vi "Main Engine.vi"(8 "error in":errorcluster) -> (0 "error out":errorcluster)   [LabVIEW 2021]
doc: "This VI will launch all engines handle and close all references.\n\n\n\nAll Rights Reserved © 2023 SyncSols"
uses:
  Controls/Main Engine State Machine Data Cluster.ctl
  Controls/Main Engine Hardware Info Data Cluster.ctl
  Controls/Main Engine DAQ Device Info.ctl
  Controls/Main Engine Serial Card Details.ctl
  Controls/Main Engine Hardware Loop Data.ctl
  Controls/Main Engine Command Cluster.ctl
  Controls/Main Engine TCP Command Data.ctl
  Controls/Main Engine Q Driver Options.ctl
  Controls/Main Engine State Machine Cases.ctl
  Controls/Main Engine Q Option.ctl
  Controls/RT-Queue's FGV Action.ctl
  Host-DQMH/Configuration/All Interface Data.ctl
  Host-DQMH/Configuration/DO Channel's.ctl
  Host-DQMH/Configuration/Analog Input Single Channel Data--Cluster.ctl
  Host-DQMH/Configuration/Config-Channel Type.ctl
  Host-DQMH/Configuration/Channel Sub-Type.ctl
  Analog Output/Controls/AO Timing Cluster.ctl
  Controls/Main Engine Engine No.Options.ctl
  Controls/Main Engine CPU Info.ctl
  Host-Control's/TCP Tx-Rx cluster.ctl
  Controls/Main Engine CPU JSON.ctl
  Controls/Main Engine Q Cluster.ctl
  <vilib>/nisyscfg/Close (System).vi
  TCP Engine/TCP Engine.lvlib
  <resource>/objmgr/nicriosae.rc
  <vilib>/NI_Real-Time Target Support.lvlib
  Host-DQMH/Configuration/Configuration.lvlib
  RT-DQMH-Module's/RT-TDMS-Logging/RT-TDMS-Logging.lvlib
  RT-DQMH-Module's/RT-AutoSequence/RT-AutoSequence.lvlib
  <vilib>/nisyscfg/nisyscfg.lvlib
  <vilib>/addons/_JKI.lib/Serialization/JSON/JKI JSON Serialization.lvlib
panel:
  out "Hardware Info 2":T1[](array[typedef]) {"Is Present?" items=["Initializing"=-2, "Unknown"=-1, "Not Present"=0, "Present"=1]}
  out "DAQ Device Info 2":T2[](array[typedef])
  out "Element's Inside the Q":i32[](array[numeric])
  out "Q-Name's":string[](array[string])
  in  "stop":bool
  in  "Start":bool
  out "LED":bool
  in  "Data Cluster":T3={"IP Address"="", "Hardware Info"=[], "Main Engine Response Q"=refnum, "Bin File Refnum"=refnum, "TCP Engine Response Q"=refnum, "TCP Engine Refnum"=refnum, "DAQ Device Info"=[], "Serial Device Info"=[], "Hardware Info Notifier"=refnum, "Main Engine Command Q"=refnum, "Variant Data"=variant, "Engine Name"="Slot5_6551_AO", "Interface"="AO", "SubCmd"="", "Serial Mode"="", "Serial Engine Reference"=[], "PLL Locked?"=FALSE, "PLL Status"="", "Ethernet Mode"=0, "Eth TCP Engine Ref"=[], "Ethernet IP Address"=[], "CPU Load"=FALSE, "Sys Session "="", "Sys Ref"=refnum, "Current time"=timestamp(0 s since 1904-01-01), "CPU Frequency"=0.0, "RT-All Q Ref"=[], "DAQ-Engine Ref"=[], "Main Engine Logging File Path"=path ""} {"Hardware Info"."Is Present?" items=["Initializing"=-2, "Unknown"=-1, "Not Present"=0, "Present"=1]}
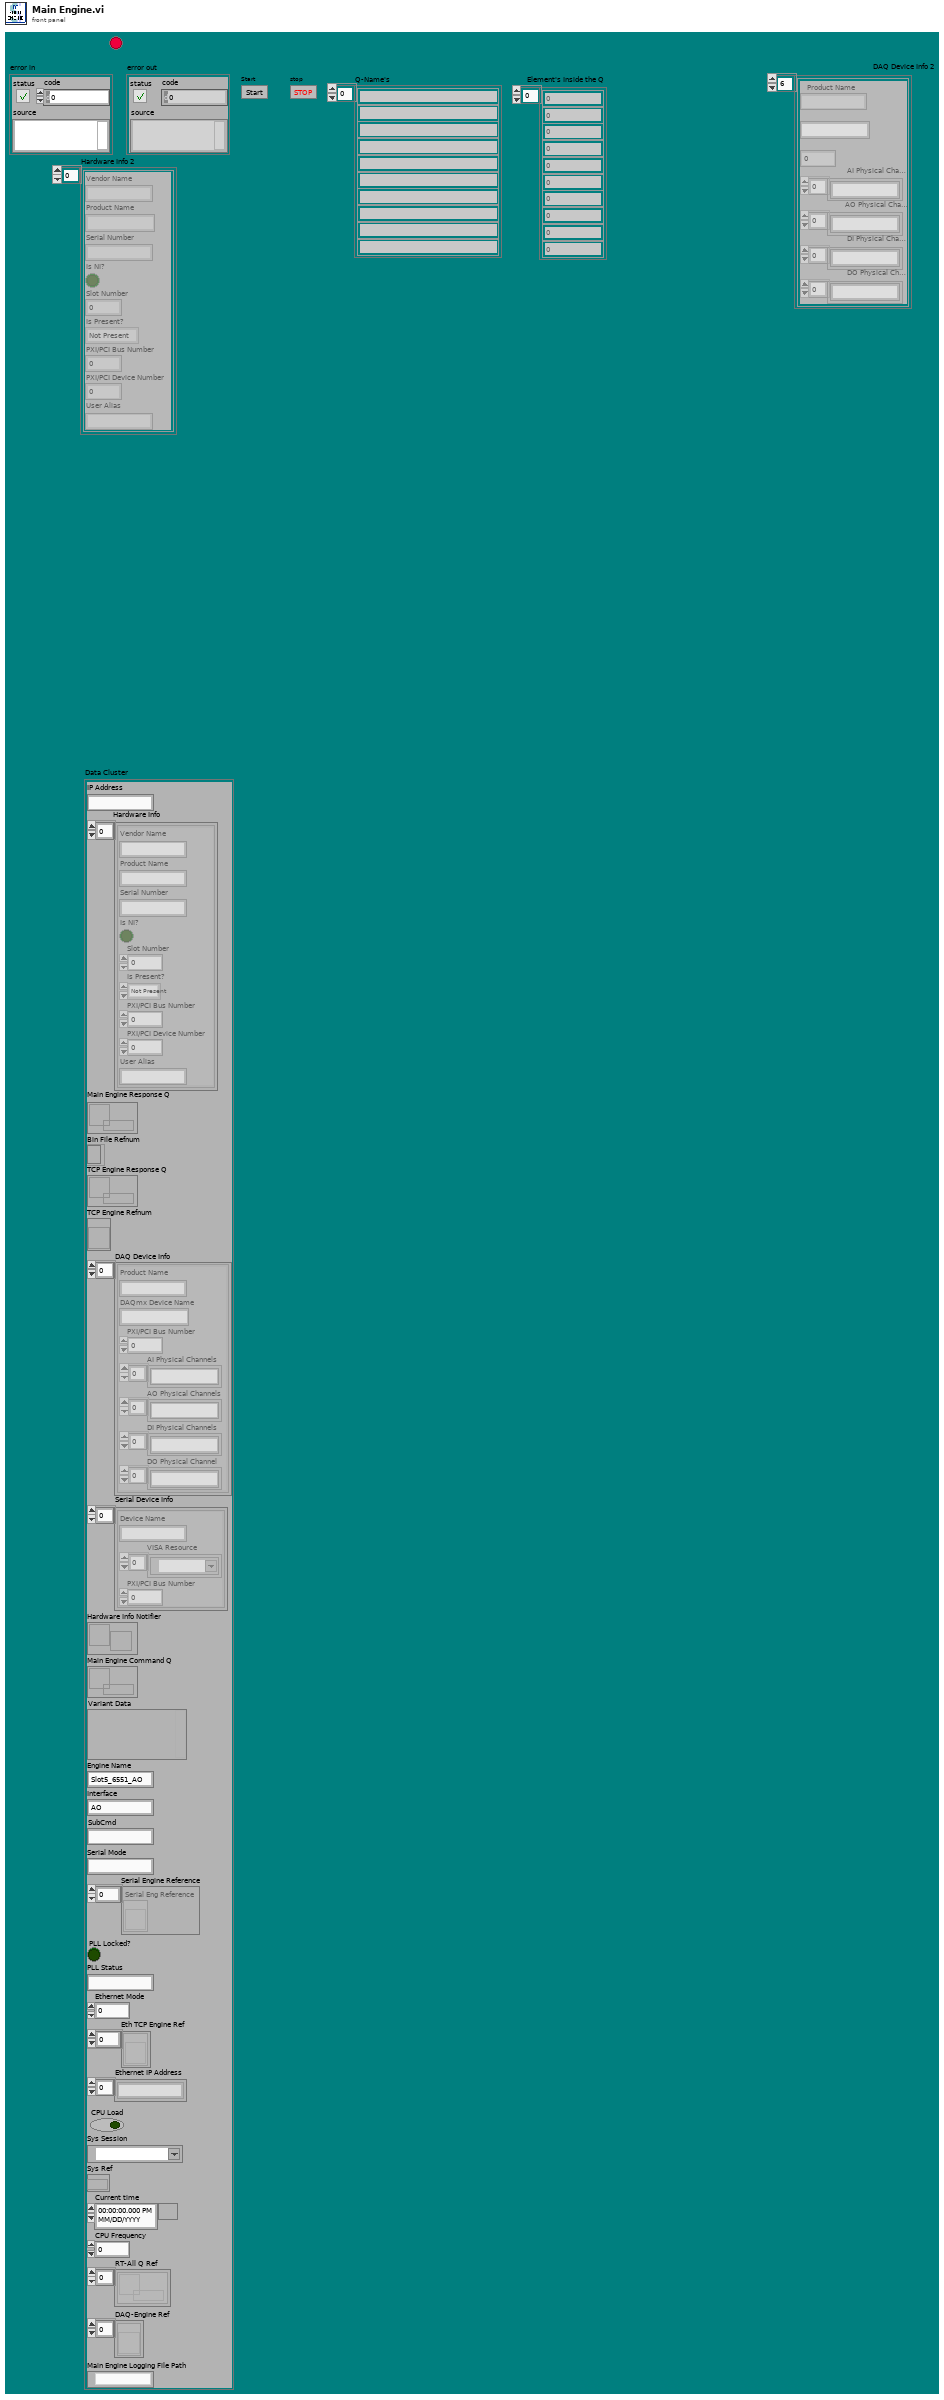
[diagram p1: front panel]
types:
  T1 = typedef "Main Engine Hardware Info Data Cluster.ctl" = cluster{"Vendor Name":string, "Product Name":string, "Serial Number":string, "Is NI?":bool, "Slot Number":i32, "Is Present?":i32, "PXI/PCI Bus Number":u32, "PXI/PCI Device Number":u32, "User Alias":string}
  T2 = typedef "Main Engine DAQ Device Info.ctl" = cluster{"Product Name":string, "DAQmx Device Name":string, "PXI/PCI Bus Number":u32, "AI Physical Channels":string[], "AO Physical Channels":string[], "DI Physical Channels":string[], "DO Physical Channel":string[]}
  T3 = typedef "Main Engine State Machine Data Cluster.ctl" = cluster{"IP Address":string, "Hardware Info":T1[], "Main Engine Response Q":refnum<queue>, "Bin File Refnum":refnum<file>, "TCP Engine Response Q":refnum<queue>, "TCP Engine Refnum":refnum<vi>, "DAQ Device Info":T2[], "Serial Device Info":T4[], "Hardware Info Notifier":refnum<notifier>, "Main Engine Command Q":refnum<queue>, "Variant Data":variant, "Engine Name":string, "Interface":string, "SubCmd":string, "Serial Mode":string, "Serial Engine Reference":refnum<vi>[], "PLL Locked?":bool, "PLL Status":string, "Ethernet Mode":u8, "Eth TCP Engine Ref":refnum<vi>[], "Ethernet IP Address":string[], "CPU Load":bool, "Sys Session ":refnum<k21>, "Sys Ref":refnum<k20>, "Current time":timestamp, "CPU Frequency":dbl, "RT-All Q Ref":refnum<queue>[], "DAQ-Engine Ref":refnum<vi>[], "Main Engine Logging File Path":path}
  T4 = typedef "Main Engine Serial Card Details.ctl" = cluster{"Device Name":string, "VISA Resource":refnum<visa-resource-name>[], "PXI/PCI Bus Number":u32}
  T5 = typedef "Configuration.lvlib/All Interface Data.ctl" = cluster{"DI Config Data":T6, "DO Config Data":T6, "AI Config Data's":cluster{"Module Name":string, "AI Channel's Data":T7[], "Analog Input Timing":T10}[]}
  T6 = typedef "Configuration.lvlib/DO Channel's.ctl" = cluster{"Channel Name":string, "Identification Name":string, "Data":u8[], "Enabled?":bool}[]
  T7 = typedef "Configuration.lvlib/Analog Input Single Channel Data--Cluster.ctl" = cluster{"Channel Name":string, "Identification Name":string, "Channel Type":T8, "Sub-Type":T9, "Data":string, "Enabled?":bool}
  T8 = typedef "Configuration.lvlib/Config-Channel Type.ctl" = enum16{"Voltage", "Current", "Thermocouple", "Acclerometer"}
  T9 = typedef "Configuration.lvlib/Channel Sub-Type.ctl" = enum16{"None", "Pressure", "Force"}
  T10 = typedef "AO Timing Cluster.ctl" = cluster{"samples per channel":i32, "sample mode":i32, "Sampling Rate":dbl}
  T11 = typedef "RT-Queue's FGV Action.ctl" = enum16{"Create Q's", "Get a Q Ref", "Get All Q Ref", "Release All Q"}
  T12 = typedef "Main Engine Q Option.ctl" = enum16{"Init", "Get"}
  T13 = typedef "Main Engine Hardware Loop Data.ctl" = cluster{"Start TCP Engine":bool, "IP Address":string, "Hardware Info":T1[]}
  T14 = typedef "Main Engine State Machine Cases.ctl" = enum16{">Poll", ".........State Machine.........", ">Init", ">Error", ">Exit", "..........MATSYA Main Engine..........", ">Init Data Communication", ">CPU Load", ">Launch All Modules", ">Write Response to Bin file", ">Get Command", ">Wait & Close All Engine"}
  T15 = typedef "Main Engine Q Driver Options.ctl" = enum16{"Initialize", "EnQ", "DeQ", "EnQ at Opp", "Get Q Status", "Flush Q", "Release Q"}
  T16 = enum16{"open", "replace", "create", "open or create", "replace or create", "replace or create with confirmation"}
  T17 = typedef "Main Engine Engine No.Options.ctl" = enum16{"Init", "Update", "Response", "Get"}
  T18 = typedef "Main Engine Command Cluster.ctl" = cluster{"State":T19, "Interface":string, "Engine Name":string, "Varient Data":variant, "SubCmd":string, "Serial Mode":string, "ARINC Board":u8, "Ethernet Mode":u8, "CPU Frequency":dbl}
  T19 = typedef "Main Engine TCP Command Data.ctl" = enum16{"Get HW Info", "Launch Module", "Get CPU Load", "Close CPU Load", "Exit"}
  T20 = typedef "TCP Tx-Rx cluster.ctl" = cluster{"Interface":string, "Command":string, "SubCmd":string, "Data":variant}
  T21 = typedef "Main Engine CPU Info.ctl" = cluster{"Total Load":u32[], "Interrupt Load":u32[], "Total Physical":dbl, "Free Physical":dbl, "Primary Disk Capacity":dbl, "Primary Disk Free":dbl}
  T22 = enum16{"big-endian, network order", "native, host order", "little-endian"}
  T23 = typedef "Main Engine Q Cluster.ctl" = cluster{"Main Engine Response Q":refnum<queue>, "TCP Engine Response Q":refnum<queue>}
  T24 = typedef "Main Engine CPU JSON.ctl" = cluster{"Interface":string, "Interface Data":cluster{"Command":string, "SubCmd":string, "Data":T21, "CPU Frequency":dbl}}
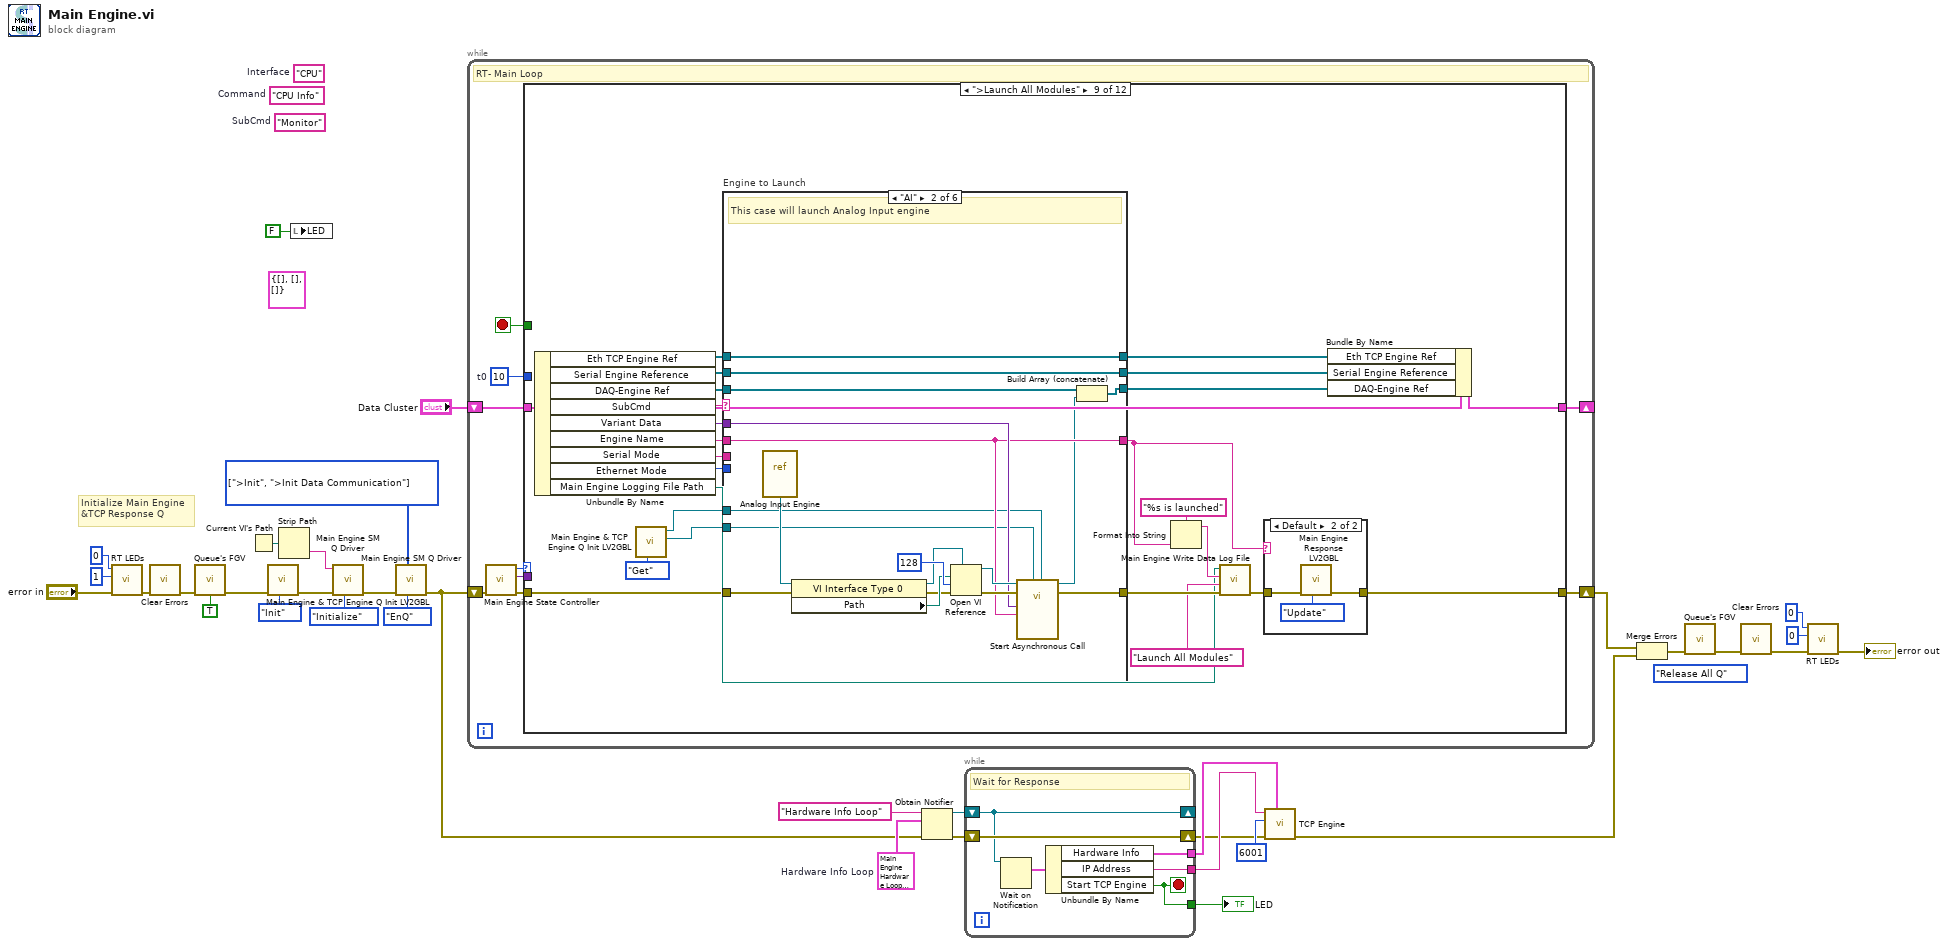
[diagram p0: block diagram]
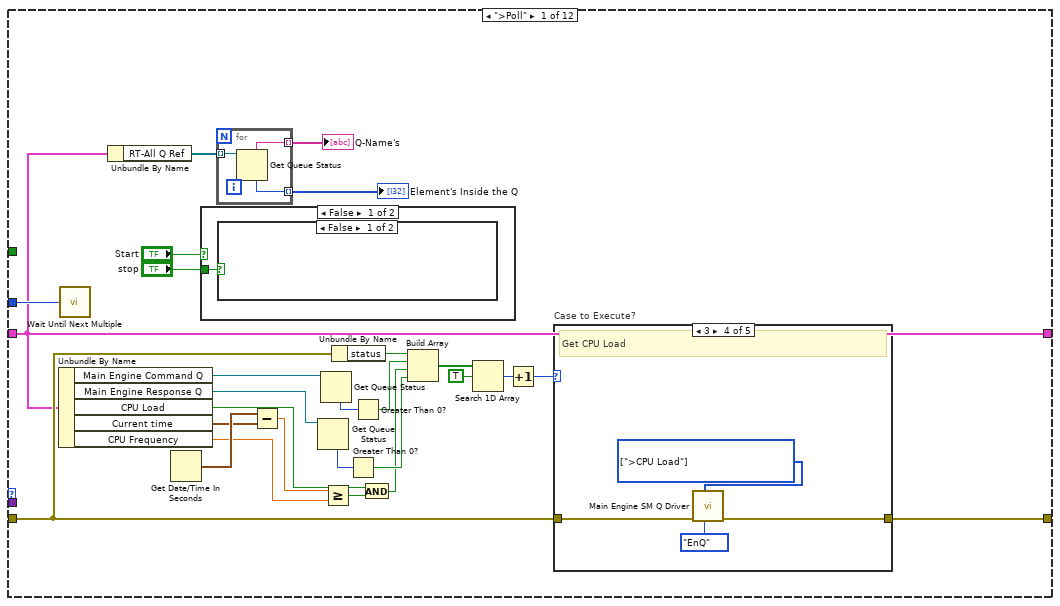
[diagram p2: hidden frame]
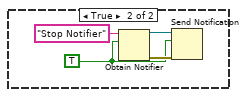
[diagram p3: hidden frame]
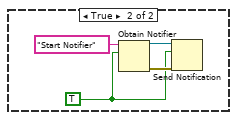
[diagram p4: hidden frame]
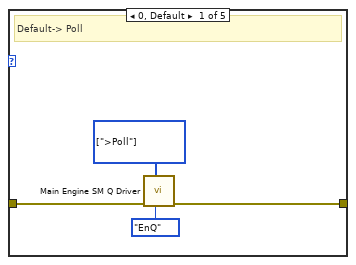
[diagram p5: hidden frame]
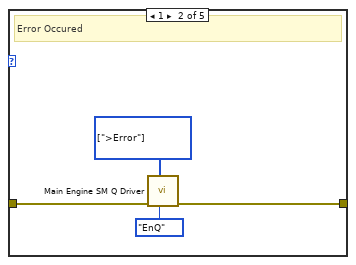
[diagram p6: hidden frame]
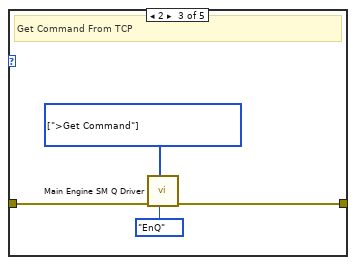
[diagram p7: hidden frame]
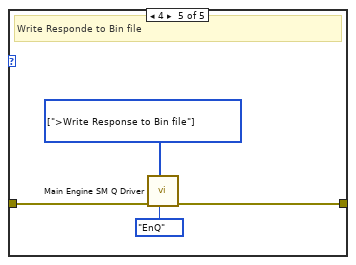
[diagram p8: hidden frame]
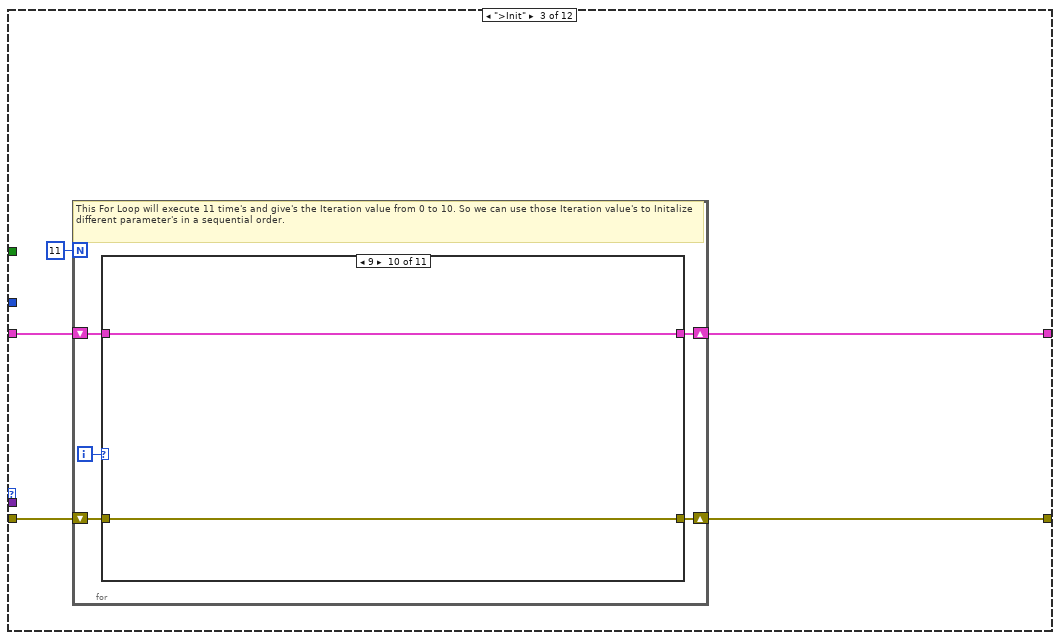
[diagram p10: hidden frame]
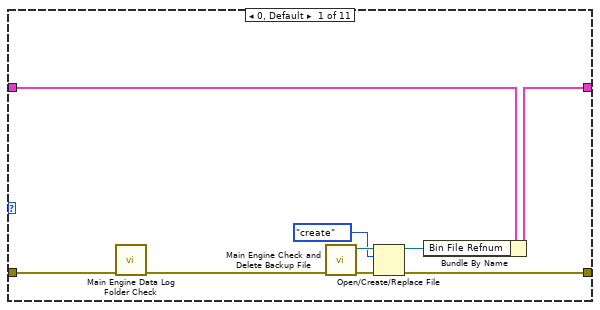
[diagram p11: hidden frame]
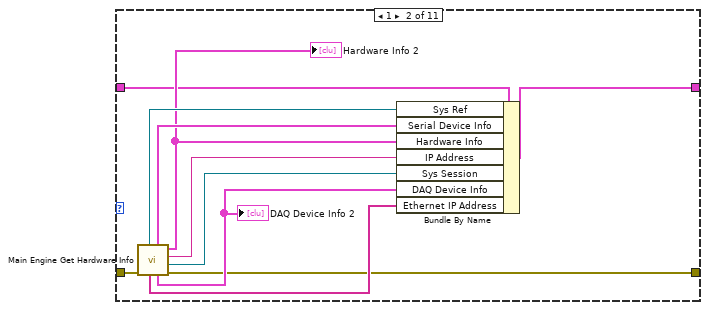
[diagram p12: hidden frame]
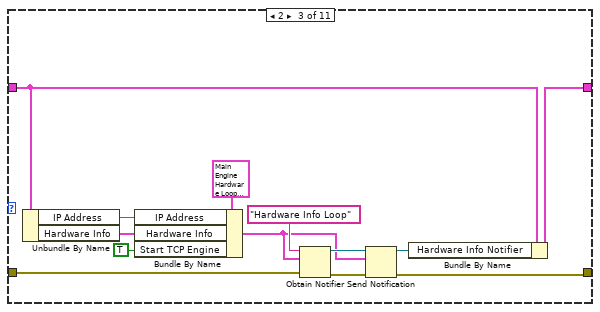
[diagram p13: hidden frame]
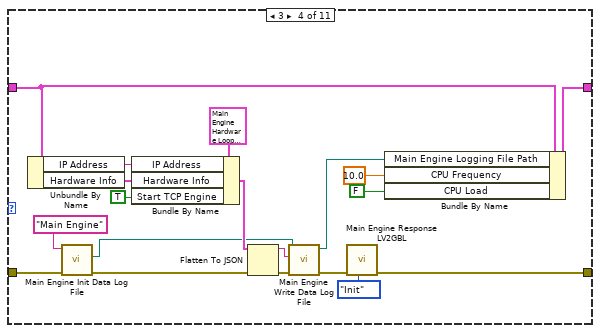
[diagram p14: hidden frame]
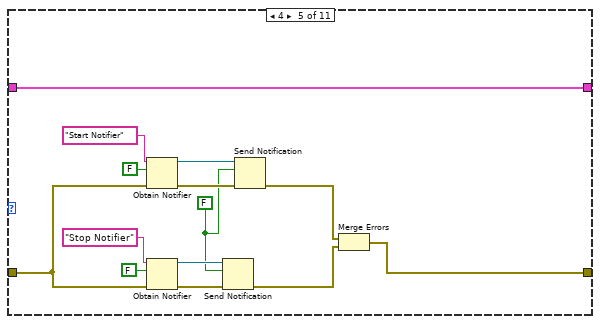
[diagram p15: hidden frame]
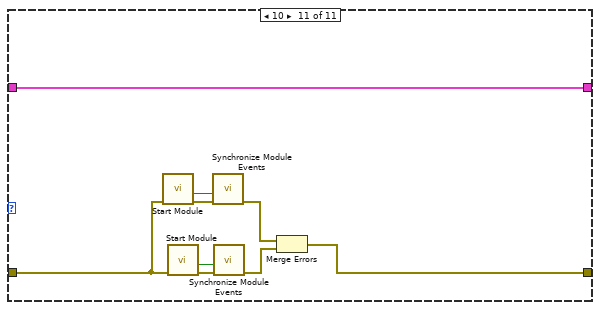
[diagram p20: hidden frame]
diagram:
  (unwired) T5 {"DI Config Data"=[], "DO Config Data"=[], "AI Config Data's"=[]} ("Interface Data")
  (unwired) "Monitor"  # SubCmd
  (unwired) "CPU Info"  # Command
  (unwired) "CPU"  # Interface
  (unwired) RT-Queue's_FGV_Action."Release All Q" ("Action")
  w24 = T13 {"Start TCP Engine"=TRUE, "IP Address"="", "Hardware Info"=[{"Vendor Name"="PXI1Slot3", "Product Name"="NI PXIe-4322", "Serial Number"="", "Is NI?"=FALSE, "Slot Number"=0, "Is Present?"=0, "PXI/PCI Bus Number"=27, "PXI/PCI Device Number"=0, "User Alias"=""}, {"Vendor Name"="PXI1Slot5", "Product Name"="NI PXI-6511", "Serial Number"="", "Is NI?"=FALSE, "Slot Number"=0, "Is Present?"=0, "PXI/PCI Bus Number"=24, "PXI/PCI Device Number"=0, "User Alias"=""}, {"Vendor Name"="PXI1Slot12", "Product Name"="NI PXIe-2727", "Serial Number"="", "Is NI?"=FALSE, "Slot Number"=0, "Is Present?"=0, "PXI/PCI Bus Number"=15, "PXI/PCI Device Number"=0, "User Alias"=""}]}  # Hardware Info Loop
  w29 = T14[] [enum.">Init", enum.">Init Data Communication"] items=[">Poll", ".........State Machine.........", ">Init", ">Error", ">Exit", "..........MATSYA Main Engine..........", ">Init Data Communication", ">CPU Load", ">Launch All Modules", ">Write Response to Bin file", ">Get Command", ">Wait & Close All Engine"]
  # "Initialize Main Engine\n&TCP Response Q"
  n1 = call <vilib>:"RT LEDs.vi"("error in (no error)"="error in", "State"=1, "LED Num"=0) -> ("error out"=w12:errorcluster)  [unwired: 3 in, 1 out]
  n2 = call <vilib>:"Clear Errors.vi"("error in (no error)"=w12) -> ("error out"=w9:errorcluster)  [unwired: 5 in, 1 out]
  n3 = call "Queue's FGV.vi"("error in"=w9, "Create new?"=TRUE) -> ("error out"=w5:errorcluster)  [unwired: 12 in, 1 out]
  n4 = Current VI's Path() -> (path=w34:path)
  n5 = call "Main Engine & TCP Engine Q Init LV2GBL.vi"("Q Option"=Main_Engine_Q_Option."Init", "error in"=w5) -> ("error out"=w4:errorcluster)  [unwired: 7 in, 2 out]
  n6 = Strip Path(path=w34) -> (name=w33:string)  [unwired: 1 out]
  n7 = local write "LED"(FALSE ("LED")) -> ()
  n8 = call "Main Engine SM Q Driver.vi"("Q Driver Options"=Main_Engine_Q_Driver_Options."Initialize", "error in"=w4, "Q Name"=w33) -> ("error out"=w31:errorcluster)  [unwired: 4 in, 4 out]
  n9 = call "Main Engine SM Q Driver.vi"("Q Driver Options"=Main_Engine_Q_Driver_Options."EnQ", "States"=w29, "error in"=w31) -> ("error out"=w6:errorcluster)  [unwired: 4 in, 4 out]
  n10 = while {
    shift-right: [w44] -> w35
    shift-left: w6 -> [w41]
    shift-right: [w42] -> _
    shift-left: "Data Cluster" -> [w36]
    stop <- w43 stop-if-true
    w37 = 10  # t0
    # "RT- Main Loop"
    n11 = call "Main Engine State Controller.vi"("error in"=w41) -> ("error out"=w40:errorcluster, "Data"=w38:variant, "SM Cases Options"=w39:T14)  [unwired: 8 in]
    n12 = case shown="\">Launch All Modules\"" w39 {
      tunnel: w40 -> [w70 w105 w107 w205 w211 w275 w286 w297 w327 w457 w499 w540]
      tunnel: [w71 w105 w106 w206 w207 w275 w276 w300 w338 w453 w486 w538] -> w44
      tunnel: [_ _ _ _ TRUE _ _ _ _ _ _ _] -> w43
      tunnel: [w48 w104 w110 w203 w209 w274 w285 w298 w344 w460 w493 w537] -> w42
      tunnel: w36 -> [w48 w104 w109 w203 w210 w274 w287 w294 w343 w460 w477 w537]
      tunnel: w38 -> [_ _ _ _ _ _ _ _ _ _ _ _]
      tunnel: w37 -> [w61 _ _ _ _ _ _ _ _ _ _ _]
      frame ">Poll" {
        n13 = Unbundle By Name(w48) -> ("Main Engine Command Q"=w51:refnum<queue>, "Main Engine Response Q"=w60:refnum<queue>, "CPU Load"=w52:bool, "Current time"=w53:timestamp, "CPU Frequency"=w54:dbl)
        n14 = call "Wait Until Next Multiple"("Count(mSec)"=w61) -> ()  [unwired: 1 out]
        n15 = Unbundle By Name(w48) -> ("RT-All Q Ref"=w47:refnum<queue>[])
        n16 = Get Date/Time In Seconds() -> (seconds since 1Jan1904=w59:timestamp)
        n17 = case shown="False" "Start" {
          tunnel: "stop" -> [w75 _]
          frame False {
            n18 = case shown="False" w75 {
              frame False {
              }
              frame True {
                w76 = TRUE
                n19 = Obtain Notifier(name (unnamed)="Stop Notifier", notification data type=w76) -> (notifier out=w77:refnum<notifier>, error out=w79:errorcluster)  [unwired: 2 in, 1 out]
                n20 = Send Notification(notification=w76, notifier=w77, error in (no error)=w79) -> ()  [unwired: 2 out]
              }
            }
          }
          frame True {
            w80 = TRUE
            n21 = Obtain Notifier(name (unnamed)="Start Notifier", notification data type=w80) -> (notifier out=w81:refnum<notifier>, error out=w83:errorcluster)  [unwired: 2 in, 1 out]
            n22 = Send Notification(notification=w80, notifier=w81, error in (no error)=w83) -> ()  [unwired: 2 out]
          }
        }
        n23 = for {
          tunnel: w47 -> [w74] mode=indexing
          tunnel: [w73] -> w46 mode=indexing
          tunnel: [w72] -> w45 mode=indexing
          n24 = Get Queue Status(queue=w74) -> (queue name=w73:string, # elements in queue=w72:i32)  [unwired: 2 in, 6 out]
        }
        "Q-Name's" <- w46
        "Element's Inside the Q" <- w45
        n25 = Subtract(x=w59, y=w53) -> (x-y=w58:dbl)
        n26 = Get Queue Status(queue=w60) -> (# elements in queue=w63:i32)  [unwired: 2 in, 7 out]
        n27 = Get Queue Status(queue=w51) -> (# elements in queue=w64:i32)  [unwired: 2 in, 7 out]
        n28 = Greater Or Equal?(x=w58, y=w54) -> (x >= y?=w56:bool)
        n29 = Unbundle By Name(w70) -> ("status"=w69:bool)
        n30 = Greater Than 0?(x=w63) -> (x > 0?=w57:bool)
        n31 = Greater Than 0?(x=w64) -> (x > 0?=w62:bool)
        n32 = And(x=w52, y=w56) -> (x .and. y?=w55:bool)
        n33 = Build Array(w69, w62, w55, w57) -> (w68:bool[])
        n34 = Search 1D Array(1D array=w68, element=TRUE) -> (index of element=w66:i32)  [unwired: 1 in]
        n35 = Increment(x=w66) -> (x+1=w65:i32)
        n36 = case "Case to Execute?" shown="3" w65 {
          tunnel: w70 -> [w85 w89 w93 w97 w101]
          tunnel: [w84 w88 w92 w96 w100] -> w71
          frame 0, Default {
            w87 = T14[] [enum.">Poll"] items=[">Poll", ".........State Machine.........", ">Init", ">Error", ">Exit", "..........MATSYA Main Engine..........", ">Init Data Communication", ">CPU Load", ">Launch All Modules", ">Write Response to Bin file", ">Get Command", ">Wait & Close All Engine"]
            # "Default-> Poll"
            n37 = call "Main Engine SM Q Driver.vi"("Q Driver Options"=Main_Engine_Q_Driver_Options."EnQ", "States"=w87, "error in"=w85) -> ("error out"=w84:errorcluster)  [unwired: 4 in, 4 out]
          }
          frame 1 {
            w90 = T14[] [enum.">Error"] items=[">Poll", ".........State Machine.........", ">Init", ">Error", ">Exit", "..........MATSYA Main Engine..........", ">Init Data Communication", ">CPU Load", ">Launch All Modules", ">Write Response to Bin file", ">Get Command", ">Wait & Close All Engine"]
            # "Error Occured"
            n38 = call "Main Engine SM Q Driver.vi"("Q Driver Options"=Main_Engine_Q_Driver_Options."EnQ", "States"=w90, "error in"=w89) -> ("error out"=w88:errorcluster)  [unwired: 4 in, 4 out]
          }
          frame 2 {
            w94 = T14[] [enum.">Get Command"] items=[">Poll", ".........State Machine.........", ">Init", ">Error", ">Exit", "..........MATSYA Main Engine..........", ">Init Data Communication", ">CPU Load", ">Launch All Modules", ">Write Response to Bin file", ">Get Command", ">Wait & Close All Engine"]
            # "Get Command From TCP"
            n39 = call "Main Engine SM Q Driver.vi"("Q Driver Options"=Main_Engine_Q_Driver_Options."EnQ", "States"=w94, "error in"=w93) -> ("error out"=w92:errorcluster)  [unwired: 4 in, 4 out]
          }
          frame 3 {
            w98 = T14[] [enum.">CPU Load"] items=[">Poll", ".........State Machine.........", ">Init", ">Error", ">Exit", "..........MATSYA Main Engine..........", ">Init Data Communication", ">CPU Load", ">Launch All Modules", ">Write Response to Bin file", ">Get Command", ">Wait & Close All Engine"]
            # "Get CPU Load"
            n40 = call "Main Engine SM Q Driver.vi"("Q Driver Options"=Main_Engine_Q_Driver_Options."EnQ", "States"=w98, "error in"=w97) -> ("error out"=w96:errorcluster)  [unwired: 4 in, 4 out]
          }
          frame 4 {
            w102 = T14[] [enum.">Write Response to Bin file"] items=[">Poll", ".........State Machine.........", ">Init", ">Error", ">Exit", "..........MATSYA Main Engine..........", ">Init Data Communication", ">CPU Load", ">Launch All Modules", ">Write Response to Bin file", ">Get Command", ">Wait & Close All Engine"]
            # "Write Responde to Bin file"
            n41 = call "Main Engine SM Q Driver.vi"("Q Driver Options"=Main_Engine_Q_Driver_Options."EnQ", "States"=w102, "error in"=w101) -> ("error out"=w100:errorcluster)  [unwired: 4 in, 4 out]
          }
        }
      }
      frame ".........State Machine........." {
      }
      frame ">Init" {
        n42 = for {
          N: 11 -> [_]
          shift-right: [w114] -> w110
          shift-left: w109 -> [w113]
          shift-right: [w111] -> w106
          shift-left: w107 -> [w112]
          i -> [w115]
          # "This For Loop will execute 11 time's and give's the Iteration value from 0 to 10. So we can use those Iteration value's to Initalize different parameter's in a sequential order."
          n43 = case shown="9" w115 {
            tunnel: [w122 w127 w137 w163 w181 w183 w185 w187 w189 w191 w200] -> w114
            tunnel: w113 -> [w123 w128 w138 w153 w181 w183 w185 w187 w189 w191 w200]
            tunnel: w112 -> [w124 w126 w141 w159 w174 w182 w184 w186 w188 w190 w192]
            tunnel: [w117 w125 w143 w166 w168 w182 w184 w186 w188 w190 w193] -> w111
            frame 0, Default {
              n44 = call "Main Engine Data Log Folder Check.vi"("error in"=w124) -> ("error out"=w118:errorcluster)  [unwired: 10 in]
              n45 = call "Main Engine Check and Delete Backup File.vi"("error in"=w118) -> ("error out"=w120:errorcluster, "Data File Path"=w121:path)  [unwired: 9 in]
              n46 = Open/Create/Replace File(file path (use dialog)=w121, error in=w120, operation (0:open)=T16."create") -> (refnum out=w116:refnum<file>, error out=w117:errorcluster)  [unwired: 3 in, 1 out]
              n47 = Bundle By Name(cluster=w123, "Bin File Refnum"=w116) -> (w122:T3)
            }
            frame 1 {
              n48 = call "Main Engine Get Hardware Info.vi"("error in"=w126) -> ("error out"=w125:errorcluster, "CPU Session"=w131:refnum<k21>, "IPAddress"=w134:string, "Hardware Info"=w129:T1[], "DAQ Device Info"=w130:T2[], "Serial Device Info"=w135:T4[], "Ethernet IP Address"=w133:string[], "CPU Ref"=w132:refnum<k20>)  [unwired: 3 in]
              "DAQ Device Info 2" <- w130
              "Hardware Info 2" <- w129
              n49 = Bundle By Name(cluster=w128, "Sys Ref"=w132, "Serial Device Info"=w135, "Hardware Info"=w129, "IP Address"=w134, "Sys Session"=w131, "DAQ Device Info"=w130, "Ethernet IP Address"=w133) -> (w127:T3)
            }
            frame 2 {
              n50 = Unbundle By Name(w138) -> ("IP Address"=w140:string, "Hardware Info"=w139:T1[])
              n51 = Bundle By Name(cluster=T13 {"Start TCP Engine"=TRUE, "IP Address"="", "Hardware Info"=[{"Vendor Name"="PXI1Slot3", "Product Name"="NI PXIe-4322", "Serial Number"="", "Is NI?"=FALSE, "Slot Number"=0, "Is Present?"=0, "PXI/PCI Bus Number"=27, "PXI/PCI Device Number"=0, "User Alias"=""}, {"Vendor Name"="PXI1Slot5", "Product Name"="NI PXI-6511", "Serial Number"="", "Is NI?"=FALSE, "Slot Number"=0, "Is Present?"=0, "PXI/PCI Bus Number"=24, "PXI/PCI Device Number"=0, "User Alias"=""}, {"Vendor Name"="PXI1Slot12", "Product Name"="NI PXIe-2727", "Serial Number"="", "Is NI?"=FALSE, "Slot Number"=0, "Is Present?"=0, "PXI/PCI Bus Number"=15, "PXI/PCI Device Number"=0, "User Alias"=""}]}, "IP Address"=w140, "Hardware Info"=w139, "Start TCP Engine"=TRUE ("Get Hard Ware Info")) -> (w142:T13)
              n52 = Obtain Notifier(name (unnamed)="Hardware Info Loop", notification data type=w142, error in (no error)=w141) -> (notifier out=w145:refnum<notifier>, error out=w144:errorcluster)  [unwired: 1 in, 1 out]
              n53 = Send Notification(notification=w142, notifier=w145, error in (no error)=w144) -> (notifier out=w136:refnum<notifier>, error out=w143:errorcluster)
              n54 = Bundle By Name(cluster=w138, "Hardware Info Notifier"=w136) -> (w137:T3)
            }
            frame 3 {
              n55 = Unbundle By Name(w153) -> ("IP Address"=w152:string, "Hardware Info"=w151:T1[])
              n56 = call "Main Engine Init Data Log File.vi"("error in"=w159, "Engine Name"="Main Engine") -> ("error out"=w161:errorcluster, "Log File Path"=w149:path)  [unwired: 8 in]
              n57 = Bundle By Name(cluster=T13 {"Start TCP Engine"=TRUE, "IP Address"="", "Hardware Info"=[{"Vendor Name"="PXI1Slot3", "Product Name"="NI PXIe-4322", "Serial Number"="", "Is NI?"=FALSE, "Slot Number"=0, "Is Present?"=0, "PXI/PCI Bus Number"=27, "PXI/PCI Device Number"=0, "User Alias"=""}, {"Vendor Name"="PXI1Slot5", "Product Name"="NI PXI-6511", "Serial Number"="", "Is NI?"=FALSE, "Slot Number"=0, "Is Present?"=0, "PXI/PCI Bus Number"=24, "PXI/PCI Device Number"=0, "User Alias"=""}, {"Vendor Name"="PXI1Slot12", "Product Name"="NI PXIe-2727", "Serial Number"="", "Is NI?"=FALSE, "Slot Number"=0, "Is Present?"=0, "PXI/PCI Bus Number"=15, "PXI/PCI Device Number"=0, "User Alias"=""}]}, "IP Address"=w152, "Hardware Info"=w151, "Start TCP Engine"=TRUE ("Get Hard Ware Info")) -> (w154:T13)
              n58 = Flatten To JSON(anything=w154, error in (no error)=w161) -> (JSON string=w162:string, 11:w160:errorcluster)  [unwired: 1 in]
              n59 = call "Main Engine Write Data Log File.vi"("error in"=w160, "Input Data"=w162, "Log file path In"=w149) -> ("error out"=w158:errorcluster, "Log File Path Out"=w150:path)  [unwired: 7 in]
              n60 = call "Main Engine Response LV2GBL.vi"("Options"=Main_Engine_Engine_No.Options."Init", "error in"=w158) -> ("error out"=w166:errorcluster)  [unwired: 7 in, 2 out]
              n61 = Bundle By Name(cluster=w153, "Main Engine Logging File Path"=w150, "CPU Frequency"=10.0, "CPU Load"=FALSE) -> (w163:T3)
            }
            frame 4 {
              w171 = FALSE ("notification")
              n62 = Obtain Notifier(name (unnamed)="Start Notifier", notification data type=FALSE, error in (no error)=w174) -> (notifier out=w176:refnum<notifier>, error out=w175:errorcluster)  [unwired: 1 in, 1 out]
              n63 = Obtain Notifier(name (unnamed)="Stop Notifier", notification data type=FALSE, error in (no error)=w174) -> (notifier out=w172:refnum<notifier>, error out=w173:errorcluster)  [unwired: 1 in, 1 out]
              n64 = Send Notification(notification=w171, notifier=w172, error in (no error)=w173) -> (error out=w169:errorcluster)  [unwired: 1 out]
              n65 = Send Notification(notification=w171, notifier=w176, error in (no error)=w175) -> (error out=w170:errorcluster)  [unwired: 1 out]
              n66 = Merge Errors(w170, w169) -> (w168:errorcluster)
            }
            frame 5 {
            }
            frame 6 {
            }
            frame 7 {
            }
            frame 8 {
            }
            frame 9 {
            }
            frame 10 {
              n67 = call "Start Module.vi"("error in"=w192) -> ("error out"=w196:errorcluster, "Wait for Event Sync?"=w197:bool)  [unwired: 7 in, 2 out]
              n68 = call "Start Module.vi"("error in"=w192) -> ("error out"=w199:errorcluster, "Wait for Event Sync?"=w198:bool)  [unwired: 7 in, 2 out]
              n69 = call "Synchronize Module Events.vi"("error in"=w196, "Wait for Event Sync?"=w197) -> ("error out"=w195:errorcluster)  [unwired: 9 in]
              n70 = call "Synchronize Module Events.vi"("error in"=w199, "Wait for Event Sync?"=w198) -> ("error out"=w194:errorcluster)  [unwired: 9 in]
              n71 = Merge Errors(w195, w194) -> (w193:errorcluster)
            }
          }
        }
      }
      frame ">Error" {
        n72 = Unbundle By Name(w203) -> ("Main Engine Logging File Path"=w201:path)
        n73 = call "Main Engine Write Data Log File.vi"("error in"=w205, "State"="Error" ("Input Data"), "Log file path In"=w201) -> ("error out"=w204:errorcluster)  [unwired: 7 in, 1 out]
        n74 = call <vilib>:"Clear Errors.vi"("error in (no error)"=w204) -> ("error out"=w206:errorcluster)  [unwired: 5 in, 1 out]
      }
      frame ">Exit" {
        n75 = for {
          N: 11 -> [_]
          shift-right: [w214] -> w207
          shift-left: w211 -> [w215]
          shift-right: [w218] -> w209
          shift-left: w210 -> [w217]
          i -> [w219]
          n76 = call <vilib>:"Clear Errors.vi"("error in (no error)"=w215) -> ("error out"=w213:errorcluster)  [unwired: 5 in, 1 out]
          n77 = case shown="4" w219 {
            tunnel: [w227 w238 w246 w249 w261 w263 w265 w267 w269 w271 w273] -> w218
            tunnel: w217 -> [w227 w238 w246 w249 w261 w263 w265 w267 w269 w271 w273]
            tunnel: [w226 w228 w241 w250 w255 w262 w264 w266 w268 w270 w272] -> w216
            tunnel: w213 -> [w222 w229 w242 w251 w259 w262 w264 w266 w268 w270 w272]
            frame 0, Default {
              n78 = Unbundle By Name(w227) -> ("TCP Engine Response Q"=w225:refnum<queue>, "Main Engine Response Q"=w220:refnum<queue>)
              n79 = Release Queue(queue=w220, force destroy? (F)=TRUE, error in (no error)=w222) -> (error out=w221:errorcluster)  [unwired: 2 out]
              n80 = Release Queue(queue=w225, force destroy? (F)=TRUE, error in (no error)=w221) -> (error out=w226:errorcluster)  [unwired: 2 out]
            }
            frame 1 {
              w230 = TRUE
              n81 = Obtain Notifier(name (unnamed)="Start Notifier", notification data type=w230, error in (no error)=w229) -> (notifier out=w236:refnum<notifier>, error out=w235:errorcluster)  [unwired: 1 in, 1 out]
              n82 = Release Notifier(notifier=w236, error in (no error)=w235) -> (error out=w232:errorcluster)  [unwired: 1 in, 2 out]
              n83 = Obtain Notifier(name (unnamed)="Stop Notifier", notification data type=w230, error in (no error)=w232) -> (notifier out=w234:refnum<notifier>, error out=w231:errorcluster)  [unwired: 1 in, 1 out]
              n84 = Release Notifier(notifier=w234, error in (no error)=w231) -> (error out=w228:errorcluster)  [unwired: 1 in, 2 out]
            }
            frame 2 {
              n85 = Unbundle By Name(w246) -> ("Hardware Info Notifier"=w239:refnum<notifier>, "Bin File Refnum"=w240:refnum<file>)
              n86 = Close File(refnum=w240, error in=w242) -> (error out=w244:errorcluster)  [unwired: 1 out]
              n87 = call "Main Engine SM Q Driver.vi"("Q Driver Options"=Main_Engine_Q_Driver_Options."Release Q", "error in"=w244) -> ("error out"=w243:errorcluster)  [unwired: 5 in, 4 out]
              n88 = Release Notifier(notifier=w239, error in (no error)=w243) -> (error out=w241:errorcluster)  [unwired: 1 in, 2 out]
            }
            frame 3 {
              n89 = Unbundle By Name(w249) -> ("Main Engine Logging File Path"=w247:path, "Sys Session"=w248:refnum<k21>)
              n90 = call-poly <vilib>:"Close.vi"("error in (no error)"=w251, "Session in"=w248) -> ("error out"=w252:errorcluster)  [unwired: 9 in]
              n91 = call "Main Engine Write Data Log File.vi"("error in"=w252, "State"="Exit", "Input Data"="Main Engine  stopped", "Log file path In"=w247) -> ("error out"=w250:errorcluster)  [unwired: 6 in, 1 out]
            }
            frame 4 {
              n92 = call "Stop Module.vi"("error in"=w259, "Wait for Module to Stop? (F)"=TRUE) -> ("error out"=w257:errorcluster)  [unwired: 9 in]
              n93 = call "Stop Module.vi"("error in"=w259, "Wait for Module to Stop? (F)"=TRUE) -> ("error out"=w256:errorcluster)  [unwired: 9 in]
              n94 = Merge Errors(w257, w256) -> (w255:errorcluster)
            }
            frame 5 {
            }
            frame 6 {
            }
            frame 7 {
            }
            frame 8 {
            }
            frame 9 {
            }
            frame 10 {
            }
          }
          n95 = call <vilib>:"Clear Errors.vi"("error in (no error)"=w216) -> ("error out"=w214:errorcluster)  [unwired: 5 in, 1 out]
        }
      }
      frame "..........MATSYA Main Engine.........." {
      }
      frame ">Init Data Communication" {
        # "This case will create the Main Engine Response queue ,TCP Engine Response queue\nand Main Engine command queue"
        n96 = Obtain Queue(max queue size (-1, unlimited)=1000, name (unnamed)="Main Engine Command Q", element data type=T18 {"State"=enum."Launch Module", "Interface"="AO", "Engine Name"="Slot5_6551_AO", "Varient Data"=variant(string "{"), "SubCmd"="", "Serial Mode"="", "ARINC Board"=0, "Ethernet Mode"=0, "CPU Frequency"=0.0} ("Main Engine Command Cluster"), error in (no error)=w286) -> (queue out=w281:refnum<queue>, error out=w280:errorcluster)  [unwired: 1 in, 1 out]
        n97 = call "Main Engine & TCP Engine Q Init LV2GBL.vi"("Q Option"=Main_Engine_Q_Option."Get", "error in"=w280) -> ("error out"=w276:errorcluster, "TCP Enigine Tx-Q"=w278:refnum<queue>, "Main Engine Tx-Q"=w279:refnum<queue>)  [unwired: 7 in]
        n98 = Bundle By Name(cluster=w287, "Main Engine Command Q"=w281, "Main Engine Response Q"=w279, "TCP Engine Response Q"=w278) -> (w285:T3)
      }
      frame ">CPU Load" {
        n99 = Unbundle By Name(w294) -> ("CPU Load"=w293:bool, "Current time"=w290:timestamp, "CPU Frequency"=w292:dbl, "TCP Engine Response Q"=w299:refnum<queue>, "Sys Ref"=w301:refnum<k20>)
        n100 = Get Date/Time In Seconds() -> (seconds since 1Jan1904=w288:timestamp)
        n101 = Subtract(x=w288, y=w290) -> (x-y=w296:dbl)
        n102 = Greater Or Equal?(x=w296, y=w292) -> (x >= y?=w295:bool)
        n103 = And(x=w293, y=w295) -> (x .and. y?=w291:bool)
        n104 = case shown="True" w291 {
          tunnel: w301 -> [_ w326]
          tunnel: [w303 w318] -> w300
          tunnel: w299 -> [_ w317]
          tunnel: w297 -> [w303 w312]
          tunnel: w290 -> [w302 _]
          tunnel: [w302 w311] -> w289
          tunnel: w288 -> [_ w311]
          frame False {
          }
          frame True {
            (unwired) T24 {"Interface"="CPU", "Interface Data"={"Command"="CPU Info", "SubCmd"="Monitor", "Data"={"Total Load"=[], "Interrupt Load"=[], "Total Physical"=0.0, "Free Physical"=0.0, "Primary Disk Capacity"=0.0, "Primary Disk Free"=0.0}, "CPU Frequency"=0.0}}
            n105 = property on="Property Node" class="System Hardware"(reference=w326, error in=w312) -> (error out=w305:errorcluster, "CpuLoadTotal"=w324:u32[], "CpuLoadIntr"=w323:u32[], "TotalPhysMem"=w322:dbl, "FreePhysMem"=w321:dbl, "TotalDisk"=w320:dbl, "FreeDisk"=w319:dbl)  [unwired: 1 out]
            n106 = Bundle By Name(cluster=T21 {"Total Load"=[], "Interrupt Load"=[], "Total Physical"=0.0, "Free Physical"=0.0, "Primary Disk Capacity"=0.0, "Primary Disk Free"=0.0}, "Total Load"=w324, "Interrupt Load"=w323, "Total Physical"=w322, "Free Physical"=w321, "Primary Disk Capacity"=w320, "Primary Disk Free"=w319) -> (w309:T21)
            n107 = To Variant(anything=w309) -> (Variant=w308:variant)
            n108 = Bundle By Name(cluster=T20 {"Interface"="CPU", "Command"="CPU Info", "SubCmd"="Monitor", "Data"=variant} ("TCP Tx-Rx Cluster"), "Interface"="CPU", "Command"="CPU Info" ("Interface Data.Command"), "SubCmd"="Monitor" ("Interface Data.SubCmd"), "Data"=w308) -> (w307:T20)
            n109 = call <vilib>:"Flatten To JSON String.vi"("error in"=w305, "Variant"=w307) -> ("error out"=w304:errorcluster, "JSON String"=w306:string)  [unwired: 8 in]
            n110 = Enqueue Element(queue=w317, element=w306, timeout in ms (-1)=10, error in (no error)=w304) -> (error out=w318:errorcluster)  [unwired: 2 out]
          }
        }
        n111 = Bundle By Name(cluster=w294, "Current time"=w289) -> (w298:T3)
      }
      frame ">Launch All Modules" {
        n112 = Unbundle By Name(w343) -> ("Eth TCP Engine Ref"=w335:refnum<vi>[], "Serial Engine Reference"=w340:refnum<vi>[], "DAQ-Engine Ref"=w341:refnum<vi>[], "SubCmd"=w351:string, "Variant Data"=w350:variant, "Engine Name"=w346:string, "Serial Mode"=w342:string, "Ethernet Mode"=w333:u8, "Main Engine Logging File Path"=w328:path)
        n113 = call "Main Engine & TCP Engine Q Init LV2GBL.vi"("Q Option"=Main_Engine_Q_Option."Get") -> ("TCP Enigine Tx-Q"=w330:refnum<queue>, "Main Engine Tx-Q"=w331:refnum<queue>)  [unwired: 8 in, 1 out]
        n114 = case "Engine to Launch" shown="\"AI\"" w351 {
          tunnel: w327 -> [w360 w365 w382 w400 w421 w433]
          tunnel: [w360 w375 w393 w411 w432 w439] -> w349
          tunnel: w350 -> [_ w374 w392 w410 w431 w438]
          tunnel: w346 -> [_ w373 w391 w409 w420 w437]
          tunnel: ["Undefined" ("Engine Name") w373 w391 w409 w420 w437] -> w337
          tunnel: w342 -> [_ _ _ _ _ _]
          tunnel: w341 -> [w357 w371 w388 w406 w428 w436]
          tunnel: [w357 w372 w389 w407 w429 w436] -> w329
          tunnel: w340 -> [w358 w370 w387 w405 w427 w435]
          tunnel: [w358 w370 w387 w405 w427 w435] -> w336
          tunnel: [w356 w369 w386 w404 w426 w434] -> w334
          tunnel: w335 -> [w356 w369 w386 w404 w426 w434]
          tunnel: w333 -> [_ _ _ _ _ _]
          tunnel: w331 -> [_ w363 w380 w398 w415 _]
          tunnel: w330 -> [_ w362 w379 w397 w416 _]
          frame Default {
            # "This case will not launch any engine"
          }
          frame "AI" {
            # "This case will launch Analog Input engine"
            n115 = vi-ref "Analog Input Engine.vi"() -> (w364:refnum<vi>)
            n116 = property class="VI Interface Type 0"(reference=w364, error in=w365) -> (reference out=w367:refnum<vi>, error out=w366:errorcluster, "Path"=w368:path)
            n117 = Open VI Reference(type specifier VI Refnum (for type only)=w367, vi path=w368, options=128, error in (no error)=w366) -> (vi reference=w377:refnum<vi>, error out=w376:errorcluster)  [unwired: 2 in]
            n118 = call-by-ref "Start Asynchronous Call"(reference=w377, error in=w376, "Main Engine Q"=w363, "TCP Enigine Q"=w362, "Engine Name"=w373, "Varient Data"=w374) -> (reference out=w361:refnum<vi>, error out=w375:errorcluster)  [unwired: 7 in, 1 out]
            n119 = Build Array (concatenate)(w371, w361) -> (w372:refnum<vi>[])
          }
          frame "AO" {
            # "This case will launch Analogl Output engine"
            n120 = vi-ref "Analog Output Engine.vi"() -> (w381:refnum<vi>)
            n121 = property class="VI Interface Type 0"(reference=w381, error in=w382) -> (reference out=w384:refnum<vi>, error out=w383:errorcluster, "Path"=w385:path)
            n122 = Open VI Reference(type specifier VI Refnum (for type only)=w384, vi path=w385, options=128, error in (no error)=w383) -> (vi reference=w395:refnum<vi>, error out=w394:errorcluster)  [unwired: 2 in]
            n123 = call-by-ref "Start Asynchronous Call"(reference=w395, error in=w394, "Main Engine Q"=w380, "TCP Enigine Q"=w379, "Engine Name"=w391, "Varient Data"=w392) -> (reference out=w390:refnum<vi>, error out=w393:errorcluster)  [unwired: 7 in, 1 out]
            n124 = Build Array (concatenate)(w388, w390) -> (w389:refnum<vi>[])
          }
          frame "DI" {
            # "This case will launch Digital Input engine"
            n125 = vi-ref "Digital Input Engine.vi"() -> (w399:refnum<vi>)
            n126 = property class="VI Interface Type 0"(reference=w399, error in=w400) -> (reference out=w402:refnum<vi>, error out=w401:errorcluster, "Path"=w403:path)
            n127 = Open VI Reference(type specifier VI Refnum (for type only)=w402, vi path=w403, options=128, error in (no error)=w401) -> (vi reference=w413:refnum<vi>, error out=w412:errorcluster)  [unwired: 2 in]
            n128 = call-by-ref "Start Asynchronous Call"(reference=w413, error in=w412, "Main Engine Q"=w398, "TCP Enigine Q"=w397, "Engine Name"=w409, "Varient Data"=w410) -> (reference out=w408:refnum<vi>, error out=w411:errorcluster)  [unwired: 7 in, 1 out]
            n129 = Build Array (concatenate)(w406, w408) -> (w407:refnum<vi>[])
          }
          frame "DO" {
            # "This case will launch Digital Output engine"
            n130 = vi-ref "Digital Output Engine.vi"() -> (w425:refnum<vi>)
            n131 = property class="VI Interface Type 0"(reference=w425, error in=w421) -> (reference out=w423:refnum<vi>, error out=w422:errorcluster, "Path"=w424:path)
            n132 = Open VI Reference(type specifier VI Refnum (for type only)=w423, vi path=w424, options=128, error in (no error)=w422) -> (vi reference=w418:refnum<vi>, error out=w417:errorcluster)  [unwired: 2 in]
            n133 = call-by-ref "Start Asynchronous Call"(reference=w418, error in=w417, "Main Engine Q"=w415, "TCP Enigine Q"=w416, "Engine Name"=w420, "Varient Data"=w431) -> (reference out=w430:refnum<vi>, error out=w432:errorcluster)  [unwired: 7 in, 1 out]
            n134 = Build Array (concatenate)(w428, w430) -> (w429:refnum<vi>[])
          }
          frame "Async" {
            # "This case will launch Asynchronous serial communication engine"
            n135 = disable-structure shown="Enabled" {
              disable-tunnel: [w448 w452] -> w439
              disable-tunnel: w438 -> [w447 _]
              disable-tunnel: w437 -> [w446 _]
              disable-tunnel: [w445 _] -> _
              disable-tunnel: w433 -> [w441 w452]
              frame Disabled {
                n136 = vi-ref "Async Serial Engine.vi"() -> (w440:refnum<vi>)
                n137 = property class="VI Interface Type 1"(reference=w440, error in=w441) -> (reference out=w443:refnum<vi>, error out=w442:errorcluster, "Path"=w444:path)
                n138 = Open VI Reference(type specifier VI Refnum (for type only)=w443, vi path=w444, options=128, error in (no error)=w442) -> (vi reference=w450:refnum<vi>, error out=w449:errorcluster)  [unwired: 2 in]
                n139 = call-by-ref "Start Asynchronous Call"(reference=w450, error in=w449, "Engine Name"=w446, "Varient Data"=w447) -> (reference out=w445:refnum<vi>, error out=w448:errorcluster)  [unwired: 9 in, 1 out]
              }
              frame Enabled {
              }
            }
          }
        }
        n140 = Format Into String(format string="%s is launched" ("Input Data"), w337) -> (resulting string=w345:string)  [unwired: 2 in, 1 out]
        n141 = call "Main Engine Write Data Log File.vi"("error in"=w349, "State"="Launch All Modules", "Input Data"=w345, "Log file path In"=w328) -> ("error out"=w339:errorcluster)  [unwired: 6 in, 1 out]
        n142 = case shown="Default" w337 {
          tunnel: w339 -> [w352 w355]
          tunnel: [w352 w354] -> w338
          frame "Undefined" {
          }
          frame Default {
            n143 = call "Main Engine Response LV2GBL.vi"("Options"=Main_Engine_Engine_No.Options."Update", "error in"=w355) -> ("error out"=w354:errorcluster)  [unwired: 7 in, 2 out]
          }
        }
        n144 = Bundle By Name(cluster=w343, "Eth TCP Engine Ref"=w334, "Serial Engine Reference"=w336, "DAQ-Engine Ref"=w329) -> (w344:T3)
      }
      frame ">Write Response to Bin file" {
        # "This Case writes  all engine response to BIN file"
        n145 = Unbundle By Name(w460) -> ("Bin File Refnum"=w459:refnum<file>, "Main Engine Response Q"=w458:refnum<queue>)
        n146 = Flush Queue(queue=w458, error in (no error)=w457) -> (remaining elements=w456:string[], error out=w455:errorcluster)  [unwired: 1 out]
        n147 = disable-structure shown="Enabled" {
          disable-tunnel: w459 -> [w464 _]
          disable-tunnel: w456 -> [w463 _]
          disable-tunnel: w455 -> [w462 w470]
          disable-tunnel: [w461 w470] -> w454
          frame Disabled {
            n148 = for {
              tunnel: w464 -> [w469]
              tunnel: w463 -> [w468] mode=indexing
              tunnel: w462 -> [w466]
              tunnel: [w465] -> w461 mode=indexing
              n149 = Write to Binary File(file (use dialog)=w469, data=w468, error in=w466, 9:T22."little-endian" ("byte order (0:big-endian, network order)")) -> (error out=w465:errorcluster)  [unwired: 2 in, 2 out]
            }
          }
          frame Enabled {
          }
        }
        n150 = Merge Errors(w454) -> (w453:errorcluster)
      }
      frame ">Get Command" {
        # "This case get data from  TCP Engine and give necessary data to respective engines"
        n151 = Unbundle By Name(w477) -> ("Main Engine Command Q"=w492:refnum<queue>, "CPU Frequency"=w472:dbl, "DAQ Device Info"=w480:T2[], "Main Engine Response Q"=w479:refnum<queue>, "TCP Engine Response Q"=w495:refnum<queue>, "Serial Device Info"=w497:T4[], "Ethernet IP Address"=w478:string[], "CPU Load"=w476:bool, "Main Engine Logging File Path"=w471:path)  [unwired: 1 out]
        n152 = Dequeue Element(queue=w492, timeout in ms (-1)=0, error in (no error)=w499) -> (element=w494:T18, error out=w496:errorcluster)  [unwired: 2 out]
        n153 = Unbundle By Name(w494) -> ("Ethernet Mode"=w481:u8, "Varient Data"=w491:variant, "Engine Name"=w490:string, "Interface"=w489:string, "SubCmd"=w488:string, "Serial Mode"=w483:string, "State"=w482:T19, "CPU Frequency"=w474:dbl)
        n154 = case "Command?" shown="\"Get HW Info\", Default" w482 {
          tunnel: w497 -> [w509 _ _ _ _]
          tunnel: w496 -> [w511 w517 w525 w530 w536]
          tunnel: w495 -> [w504 _ _ _ _]
          tunnel: [w510 w516 w524 w529 w536] -> w487
          tunnel: w480 -> [w507 _ _ _ _]
          tunnel: ["Hardware Info is Obtained" ("State") "Main Engine is closed" ("State") "All Modules are launched" ("State") "Get CPU Load" ("State") "Close CPU Load" ("State")] -> w484
          tunnel: w479 -> [w505 _ _ _ _]
          tunnel: w478 -> [w500 _ _ _ _]
          tunnel: w476 -> [w502 _ w520 _ _]
          tunnel: [w502 FALSE ("CPU Load") w520 TRUE ("CPU Load") FALSE ("CPU Load")] -> w475
          tunnel: w474 -> [_ _ _ w526 _]
          tunnel: [w501 w512 w519 w526 w533] -> w473
          tunnel: w472 -> [w501 w512 w519 _ w533]
          frame "Get HW Info", Default {
            n155 = Bundle By Name(cluster=T23 {"Main Engine Response Q"=refnum, "TCP Engine Response Q"=refnum} ("Cluster"), "Main Engine Response Q"=w505, "TCP Engine Response Q"=w504) -> (w503:T23)
            n156 = call "Main Engine Send Hardware Info.vi"("Q Cluster"=w503, "DAQ Device Info"=w507, "error in"=w511, "Ethernet IP Address"=w500, "Serial Device Info"=w509) -> ("error out"=w510:errorcluster)  [unwired: 6 in]
          }
          frame "Exit" {
            w515 = T14[] [enum.">Write Response to Bin file", enum.">Wait & Close All Engine", enum.">Exit"] items=[">Poll", ".........State Machine.........", ">Init", ">Error", ">Exit", "..........MATSYA Main Engine..........", ">Init Data Communication", ">CPU Load", ">Launch All Modules", ">Write Response to Bin file", ">Get Command", ">Wait & Close All Engine"] ("States")
            n157 = call "Main Engine SM Q Driver.vi"("Q Driver Options"=Main_Engine_Q_Driver_Options."EnQ", "States"=w515, "error in"=w517) -> ("error out"=w516:errorcluster)  [unwired: 4 in, 4 out]
          }
          frame "Launch Module" {
            w522 = T14[] [enum.">Launch All Modules"] items=[">Poll", ".........State Machine.........", ">Init", ">Error", ">Exit", "..........MATSYA Main Engine..........", ">Init Data Communication", ">CPU Load", ">Launch All Modules", ">Write Response to Bin file", ">Get Command", ">Wait & Close All Engine"] ("States")
            n158 = call "Main Engine SM Q Driver.vi"("Q Driver Options"=Main_Engine_Q_Driver_Options."EnQ", "States"=w522, "error in"=w525) -> ("error out"=w524:errorcluster)  [unwired: 4 in, 4 out]
          }
          frame "Get CPU Load" {
            w527 = T14[] [enum.">CPU Load"] items=[">Poll", ".........State Machine.........", ">Init", ">Error", ">Exit", "..........MATSYA Main Engine..........", ">Init Data Communication", ">CPU Load", ">Launch All Modules", ">Write Response to Bin file", ">Get Command", ">Wait & Close All Engine"] ("States")
            n159 = call "Main Engine SM Q Driver.vi"("Q Driver Options"=Main_Engine_Q_Driver_Options."EnQ", "States"=w527, "error in"=w530) -> ("error out"=w529:errorcluster)  [unwired: 4 in, 4 out]
          }
          frame "Close CPU Load" {
          }
        }
        n160 = Bundle By Name(cluster=w477, "Ethernet Mode"=w481, "Variant Data"=w491, "Engine Name"=w490, "Interface"=w489, "SubCmd"=w488, "Serial Mode"=w483, "CPU Load"=w475, "CPU Frequency"=w473) -> (w493:T3)
        n161 = call "Main Engine Write Data Log File.vi"("error in"=w487, "State"="Get Command", "Input Data"=w484, "Log file path In"=w471) -> ("error out"=w486:errorcluster)  [unwired: 6 in, 1 out]
      }
      frame ">Wait & Close All Engine" {
        # "This case will wait for response from all engines and close their references"
        n162 = while {
          shift-right: [w546] -> w539
          shift-left: w540 -> [w547]
          stop <- w543 stop-if-true
          # "Waiting for Response"
          n163 = call "Main Engine Response LV2GBL.vi"("Options"=Main_Engine_Engine_No.Options."Get", "error in"=w547) -> ("error out"=w546:errorcluster, "Response"=w544:i32, "Update"=w545:i32)  [unwired: 7 in]
          n164 = call "Wait"("Count(mSec)"=u32 100 ("milliseconds to wait")) -> ()  [unwired: 1 out]
          n165 = Equal?(x=w545, y=w544) -> (x = y?=w543:bool)
        }
        n166 = call "Main Engine All Engine Reference Close.vi"("error in"=w539, "Data Cluster"=w537) -> ("error out"=w538:errorcluster)  [unwired: 9 in]
      }
    }
  }
  n167 = Obtain Notifier(name (unnamed)="Hardware Info Loop", notification data type=w24, error in (no error)=w6) -> (notifier out=w25:refnum<notifier>, error out=w26:errorcluster)  [unwired: 1 in, 1 out]
  n168 = while {
    tunnel: [w552] -> w23
    tunnel: [w550] -> w22
    tunnel: [w549] -> w21
    shift-right: [w551] -> w19
    shift-left: w26 -> [w551]
    shift-right: [w548] -> _
    shift-left: w25 -> [w548]
    stop <- w549 stop-if-true
    # "Wait for Response"
    n169 = Wait on Notification(notifier=w548) -> (notification=w553:T13)  [unwired: 3 in, 3 out]
    n170 = Unbundle By Name(w553) -> ("Hardware Info"=w550:T1[], "IP Address"=w552:string, "Start TCP Engine"=w549:bool)
  }
  "LED" <- w21
  n171 = call "TCP Engine.vi"("Hardware Info"=w22, "error in"=w19, "Port"=u16 6001, "IP Address"=w23) -> ("error out"=w11:errorcluster)  [unwired: 7 in]
  n172 = Merge Errors(w35, w11) -> (w8:errorcluster)
  n173 = call "Queue's FGV.vi"("error in"=w8) -> ("error out"=w7:errorcluster)  [unwired: 13 in, 1 out]
  n174 = call <vilib>:"Clear Errors.vi"("error in (no error)"=w7) -> ("error out"=w10:errorcluster)  [unwired: 5 in, 1 out]
  n175 = call <vilib>:"RT LEDs.vi"("error in (no error)"=w10, "State"=0, "LED Num"=0) -> ("error out"=→"error out":errorcluster)  [unwired: 3 in, 1 out]
